vi "Read Rack Status.vi"(8 "Error In":errorcluster, 11 "KIT-QVA in":refnum<class "KIT-QVA.lvclass">) -> (0 "Error Out":errorcluster, 3 "KIT-QVA out":refnum<class "KIT-QVA.lvclass">)   [LabVIEW 2014, in "KIT-QVA.lvlib" / "KIT-QVA.lvclass"]
doc: "Read rack status and publish"
uses:
  KIT-QVA.lvclass
  KIT-QVA.lvclass/KIT-QVA.ctl
  instr.lib/KIT-QV/KIT QV.lvlib
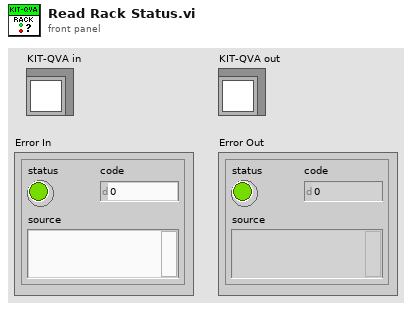
[diagram p1: front panel]
types:
  T1 = cluster{"System Test":bool, "Test Mode":bool, "Fault":bool, "Quench":bool, "U/T Fault":bool, "Bus Error":bool, "System Fault":bool, "Control Mode":bool}
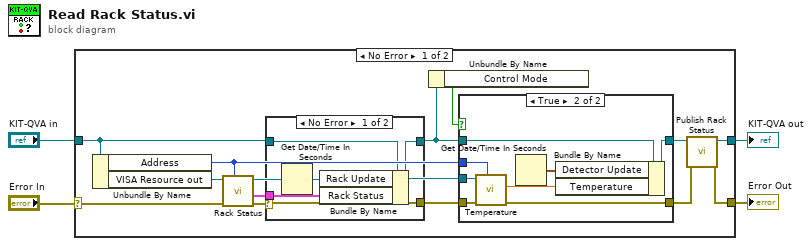
[diagram p0: block diagram]
diagram:
  n1 = case shown="No Error" "Error In" {
    selector: "Error In" -> [w17 w37]
    tunnel: [w8 w37] -> w3
    tunnel: [w9 w36] -> w1
    tunnel: "KIT-QVA in" -> [w15 w36]
    frame No Error {
      n2 = Unbundle By Name(w15) -> ("Address"=w11:u16, "VISA Resource out"=w18:refnum<visa-resource-name>)
      n3 = call "Rack Status.vi"("Address"=w11, "Error In"=w17, "VISA Resource in"=w18) -> ("Error Out"=w14:errorcluster, "Rack Status Cluster"=w16:T1, "VISA Resource out"=w13:refnum<visa-resource-name>)  [unwired: 5 in, 1 out]
      n4 = case shown="No Error" w14 {
        selector: w14 -> [w30 w34]
        tunnel: w16 -> [w33 _]
        tunnel: w15 -> [w32 w35]
        tunnel: [w31 w35] -> w6
        tunnel: [w30 w34] -> w12
        frame No Error {
          n5 = Get Date/Time In Seconds() -> (seconds since 1Jan1904=w29:timestamp)
          n6 = Bundle By Name(cluster=w32, "Rack Update"=w29, "Rack Status"=w33) -> (w31:refnum<class "KIT-QVA.lvclass">)
        }
        frame Error {
        }
      }
      n7 = Unbundle By Name(w6) -> ("Control Mode"=w5:bool)
      n8 = case shown="True" w5 {
        tunnel: w13 -> [_ w28]
        tunnel: w12 -> [w19 w27]
        tunnel: w11 -> [_ w26]
        tunnel: w6 -> [w20 w25]
        tunnel: [w20 w23] -> w10
        tunnel: [w19 w22] -> w7
        frame False {
        }
        frame True {
          n9 = call "Temperature.vi"("Address"=w26, "Error In"=w27, "VISA Resource in"=w28) -> ("Error Out"=w22:errorcluster, "Temperature"=w24:dbl[unit])  [unwired: 6 in, 1 out]
          n10 = Get Date/Time In Seconds() -> (seconds since 1Jan1904=w21:timestamp)
          n11 = Bundle By Name(cluster=w25, "Detector Update"=w21, "Temperature"=w24) -> (w23:refnum<class "KIT-QVA.lvclass">)
        }
      }
      n12 = call "Publish Rack Status.vi"("Error In"=w7, "KIT-QVA in"=w10) -> ("Error Out"=w8:errorcluster, "KIT-QVA out"=w9:refnum<class "KIT-QVA.lvclass">)  [unwired: 8 in]
    }
    frame Error {
    }
  }
  "Error Out" <- w3
  "KIT-QVA out" <- w1
